vi "PRL ARR Calculate Ratio of True.vi"(11 "Array":bool[](array[boolean])) -> (3 "True Ratio":dbl)   [LabVIEW 2013, in "PMU Recorder Light.lvlib"]
uses:
  PMU Recorder Light.lvlib
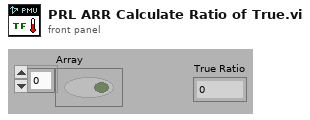
[diagram p1: front panel]
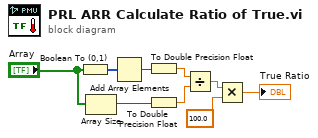
[diagram p0: block diagram]
diagram:
  n1 = Boolean To (0,1)(Boolean="Array") -> (0, 1=w5:i16[])
  n2 = Array Size(array="Array") -> (size(s)=w2:i32)
  n3 = Add Array Elements(numeric array=w5) -> (sum=w6:i16)
  n4 = To Double Precision Float(number=w6) -> (double precision float=w4:dbl)
  n5 = To Double Precision Float(number=w2) -> (double precision float=w3:dbl)
  n6 = Divide(x=w4, y=w3) -> (x/y=w7:dbl)
  n7 = Multiply(x=w7, y=100.0) -> (x*y=→"True Ratio":dbl)
